vi "Byte Buffer.Get Buffer Size.vi"(8 "error in (no error)":errorcluster, 11 "Byte Buffer in":refnum<class "Byte Buffer.lvclass">) -> (0 "error out":errorcluster, 2 "buffer size":u64, 3 "Byte Buffer out":refnum<class "Byte Buffer.lvclass">)   [LabVIEW 2016, in "VeriStand Data.lvlib" / "Byte Buffer.lvclass"]
uses:
  Byte Buffer.lvclass
  Byte Buffer.lvclass/Byte Buffer.ctl
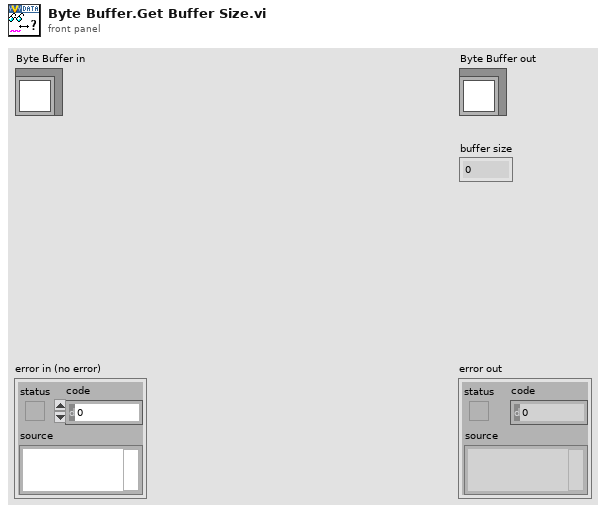
[diagram p1: front panel]
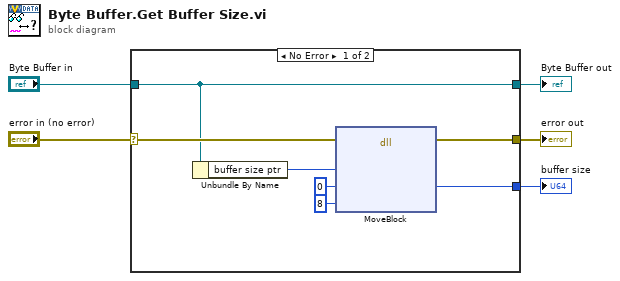
[diagram p0: block diagram]
diagram:
  n1 = case shown="No Error" "error in (no error)" {
    selector: "error in (no error)" -> [w12 w13]
    tunnel: [w10 w13] -> w4
    tunnel: [w6 w14] -> w2
    tunnel: "Byte Buffer in" -> [w6 w14]
    tunnel: [w7 _] -> w1
    frame No Error {
      n2 = Unbundle By Name(w6) -> ("buffer size ptr"=w11:u64)
      n3 = dll-call lib="LabVIEW" fn="MoveBlock"(error in=w12, "src"=w11, "dst"=u64 0 ("buffer size"), "size"=8) -> (error out=w10:errorcluster, "dst"=w7:u64)  [unwired: 5 in, 1 out]
    }
    frame Error {
    }
  }
  "error out" <- w4
  "Byte Buffer out" <- w2
  "buffer size" <- w1
